vi "Write Output Rate.vi"(8 "error in (no error)":errorcluster, 10 "Output Rate":dbl, 11 "External Clock in":refnum<class "External Clock.lvclass">) -> (0 "error out":errorcluster, 3 "External Clock out":refnum<class "External Clock.lvclass">)   [LabVIEW 2014, in "External Clock.lvclass"]
uses:
  External Clock.lvclass
  External Clock.lvclass/External Clock.ctl
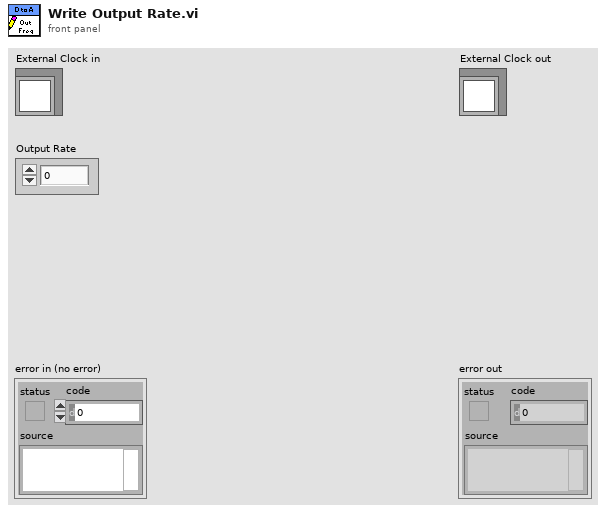
[diagram p1: front panel]
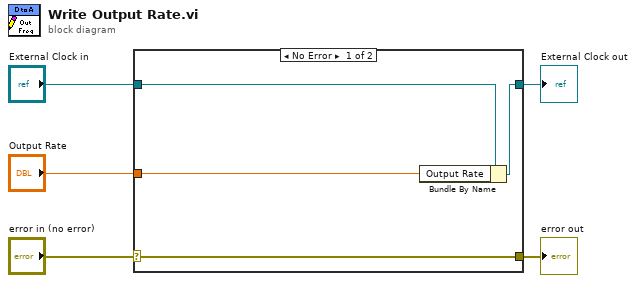
[diagram p0: block diagram]
diagram:
  n1 = case shown="No Error" "error in (no error)" {
    selector: "error in (no error)" -> [w9 w10]
    tunnel: [w9 w10] -> w4
    tunnel: [w7 w11] -> w2
    tunnel: "External Clock in" -> [w8 w11]
    tunnel: "Output Rate" -> [w6 _]
    frame No Error {
      n2 = Bundle By Name(cluster=w8, "Output Rate"=w6) -> (w7:refnum<class "External Clock.lvclass">)
    }
    frame Error {
    }
  }
  "error out" <- w4
  "External Clock out" <- w2
